vi "Test - List Devices.vi"() -> ()   [LabVIEW 2020]
uses:
  RTL-SDR/Device/Device.lvclass
panel:
  out "error out":errorcluster
  out "Devices":T1(array[cluster])
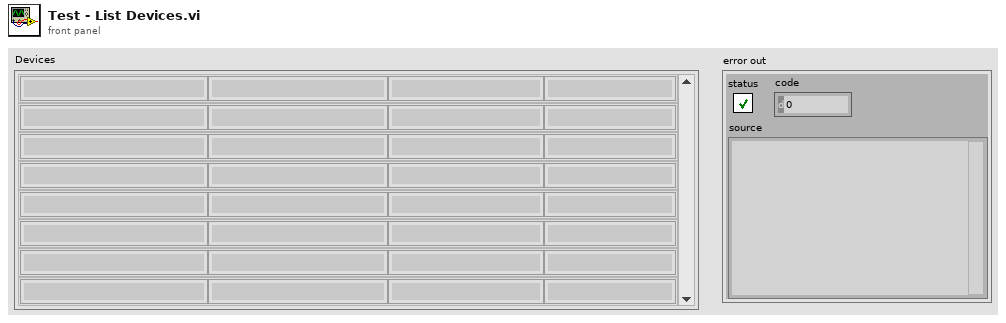
[diagram p1: front panel]
types:
  T1 = cluster{"String":string, "String 2":string, "String 3":string, "String 4":string}[]
  T2 = cluster{"Properties:Name":string, "Properties:Manufacturer":string, "Properties:Product":string, "Properties:Serial":string}
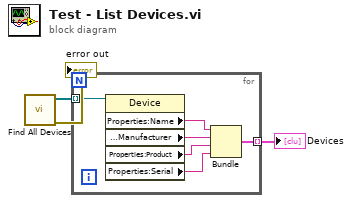
[diagram p0: block diagram]
diagram:
  n1 = call "Find All Devices.vi"() -> ("error out"=→"error out":errorcluster, "Devices"=w3:refnum<class "Device.lvclass">[])  [unwired: 10 in]
  n2 = for {
    tunnel: w3 -> [w9] mode=indexing
    tunnel: [w4] -> w2 mode=indexing
    n3 = property class="Device"(reference=w9) -> ("Properties:Name"=w5:string, "Properties:Manufacturer"=w8:string, "Properties:Product"=w7:string, "Properties:Serial"=w6:string)  [unwired: 1 in, 2 out]
    n4 = Bundle("Properties:Name"=w5, "Properties:Manufacturer"=w8, "Properties:Product"=w7, "Properties:Serial"=w6) -> (w4:T2)  [unwired: 1 in]
  }
  "Devices" <- w2
